vi "Show ROI Name Dialog.vi"(8 "error in (no error)":errorcluster, 10 "ROI Descriptor":T1 {"Contours"."Type" items=["No Selection", "Point", "Line", "Rectangle", "Oval", "Polygon", "Freehand Region", "Annulus", "Unused2", "Unused3", "Broken Line", "Freehand Line", "Rotated Rectangle"]}, 11 "IMAQ Display in":refnum<class "HIJ Vision Display.lvclass">) -> (0 "error out":errorcluster, 3 "IMAQ Display out":refnum<class "HIJ Vision Display.lvclass">)   [LabVIEW 2014, in "HIJ Vision Display.lvlib" / "HIJ Vision Display.lvclass"]
uses:
  HIJ Vision Display.lvclass
  ROI Name Dialog/Select Report File Dialog/ROI Name Dialog.lvclass
  ROI Name Dialog/Select Report File Dialog/ROI Name Dialog.lvclass/ROI Name Dialog.ctl
  <vilib>/ActorFramework/Actor/Actor.lvclass
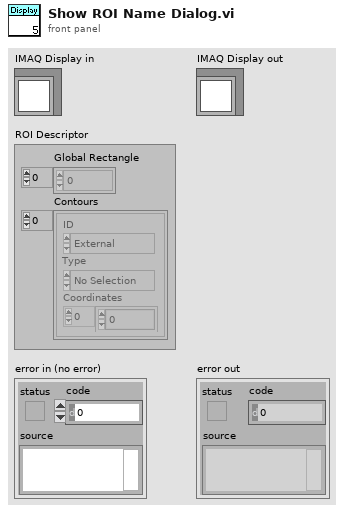
[diagram p1: front panel]
types:
  T1 = typedef "ROI Descriptor" = cluster{"Global Rectangle":i32[], "Contours":cluster{"ID":enum32{"External", "Internal"}, "Type":u32, "Coordinates":i32[]}[]}
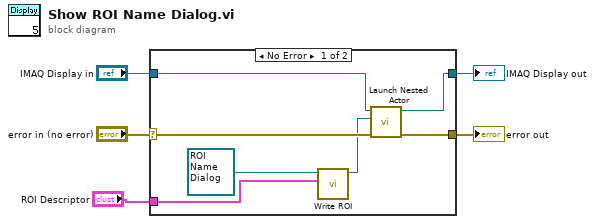
[diagram p0: block diagram]
diagram:
  n1 = case shown="No Error" "error in (no error)" {
    selector: "error in (no error)" -> [w11 w14]
    tunnel: [w10 w14] -> w4
    tunnel: [w6 w13] -> w2
    tunnel: "IMAQ Display in" -> [w12 w13]
    tunnel: "ROI Descriptor" -> [w7 _]
    frame No Error {
      n2 = call "Write ROI.vi"("ROI"=w7, "ROI Name Dialog in"=refnum<class "ROI Name Dialog.lvclass"> refnum ("ROI Name Dialog.lvlib:ROI Name Dialog.lvclass")) -> ("ROI Name Dialog out"=w8:refnum<class "ROI Name Dialog.lvclass">)  [unwired: 8 in, 1 out]
      n3 = call <vilib>:"Launch Nested Actor.vi"("error in (no error)"=w11, "Nested Actor"=w8, "Caller Actor in"=w12) -> ("error out"=w10:errorcluster, "Caller Actor out"=w6:refnum<class "HIJ Vision Display.lvclass">)  [unwired: 6 in, 1 out]
    }
    frame Error {
    }
  }
  "error out" <- w4
  "IMAQ Display out" <- w2
